vi "Write Async Message.vi"(8 "error in (no error)":errorcluster, 10 "Async Methods Actor.lvlib:Async Message.lvclass":refnum<class "Async Message.lvclass">, 11 "Completion Notification Msg in":refnum<class "Completion Notification Msg.lvclass">) -> (0 "error out":errorcluster, 3 "Completion Notification Msg out":refnum<class "Completion Notification Msg.lvclass">)   [LabVIEW 2023, in "Async Methods Actor.lvlib" / "Completion Notification Msg.lvclass"]
uses:
  Completion Notification Msg.lvclass
  Async Message/Async Message.lvclass
  C:/Program Files/National Instruments/LabVIEW 2023/vi.lib/ActorFramework/Message/Message.lvclass
  <vilib>/ActorFramework/Message/Message.lvclass
  Completion Notification Msg.lvclass/Completion Notification Msg.ctl
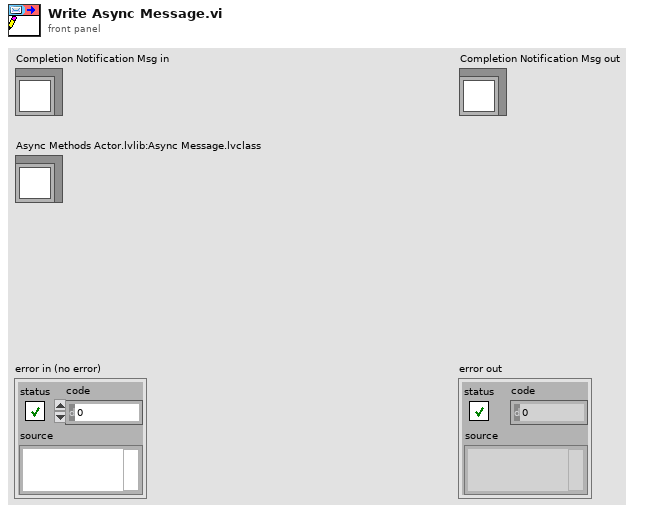
[diagram p1: front panel]
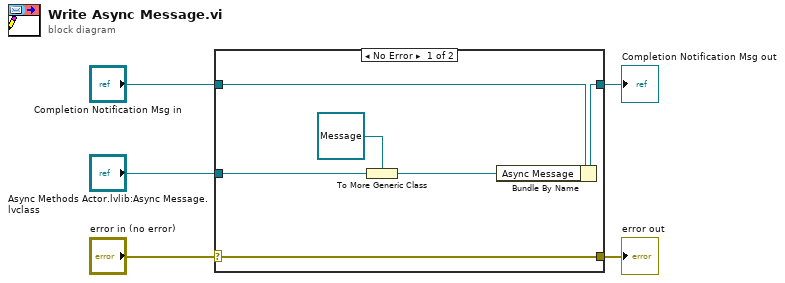
[diagram p0: block diagram]
diagram:
  n1 = case shown="No Error" "error in (no error)" {
    selector: "error in (no error)" -> [w11 w12]
    tunnel: [w11 w12] -> w4
    tunnel: [w9 w13] -> w2
    tunnel: "Completion Notification Msg in" -> [w10 w13]
    tunnel: "Async Methods Actor.lvlib:Async Message.lvclass" -> [w8 _]
    frame No Error {
      n2 = To More Generic Class(target class=refnum<class "Message.lvclass"> refnum ("Actor Framework:Message"), reference=w8) -> (generic class reference=w7:refnum<class "Message.lvclass">)
      n3 = Bundle By Name(cluster=w10, "Async Message"=w7) -> (w9:refnum<class "Completion Notification Msg.lvclass">)
    }
    frame Error {
    }
  }
  "error out" <- w4
  "Completion Notification Msg out" <- w2
